vi "get_issues_listbox_items.vi"(10 "CLZ Vol ID":string, 11 "CLZ Comics in":refnum<class "CLZ Comics.lvclass">) -> (1 "id":i32, 2 "listbox contents":string[][](array[string]), 3 "CLZ Comics out":refnum<class "CLZ Comics.lvclass">)   [LabVIEW 2024, in "CLZ_to_ComicVine.lvlib" / "CLZ Comics.lvclass"]
uses:
  CLZ Comics.lvclass
  CLZ Comics.lvclass/CLZ Comics.ctl
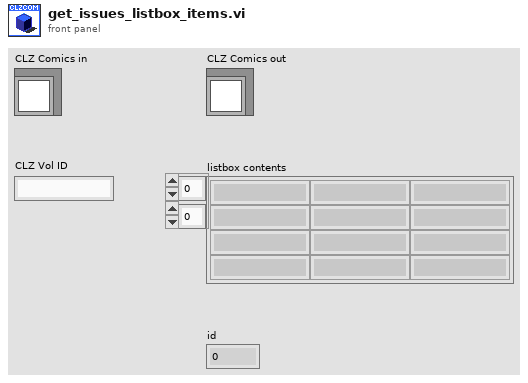
[diagram p1: front panel]
types:
  T1 = typedef "CLZ_to_ComicVine.lvlib/CLZ Comics.lvclass/volume--cluster.ctl" = cluster{"id":i32, "name":string, "issues":T2[], "matched":bool}
  T2 = typedef "CLZ_to_ComicVine.lvlib/CLZ Comics.lvclass/issue_number--cluster.ctl" = cluster{"numeric":dbl, "issue":string, "variant":string}
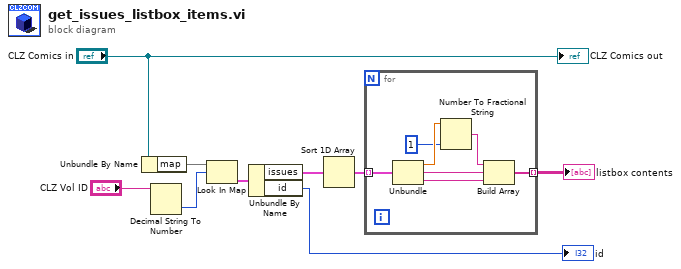
[diagram p0: block diagram]
diagram:
  n1 = Unbundle By Name("CLZ Comics in") -> ("map"=w8:map{i32, T1})
  n2 = Decimal String To Number(string="CLZ Vol ID") -> (number=w6:i32)  [unwired: 2 in, 1 out]
  n3 = Look In Map(map=w8, key=w6) -> (value=w5:T1)  [unwired: 1 in, 1 out]
  n4 = Unbundle By Name(w5) -> ("issues"=w3:T2[], "id"=→"id":i32)
  n5 = Sort 1D Array(array=w3) -> (sorted array=w4:T2[])
  n6 = for {
    tunnel: w4 -> [w16] mode=indexing
    tunnel: [w11] -> w2 mode=indexing
    n7 = Unbundle(w16) -> ("numeric"=w15:dbl, "issue"=w13:string, "variant"=w12:string)
    n8 = Number To Fractional String(number=w15, precision (6)=i16 1) -> (F-format string=w14:string)  [unwired: 2 in]
    n9 = Build Array(w14, w13, w12) -> (w11:string[])
  }
  "listbox contents" <- w2
  "CLZ Comics out" <- "CLZ Comics in"
